vi "play-AFM-raster-imaging-open-loop.vi"() -> ()   [LabVIEW 2015]
uses:
  raster-scan-params.ctl
  <vilib>/userdefined/High Color/nirio_resource_hc.ctl
  <vilib>/Utility/file.llb/Read From Spreadsheet File (DBL).vi
  <vilib>/FPGAPlugInAG/cRIO-9082/niLvFpga_Open_cRIO-9082.vi
  <vilib>/rvi/interface/common/dynamic/niFpgaDynamicAddResources.vi
  <vilib>/FPGAPlugInAG/Dynamic/niLvFpga_Reset_Dynamic.vi
  <vilib>/rvi/interface/common/niFpgaWaitOnOcc.vi
  <vilib>/Utility/error.llb/Error Cluster From Error Code.vi
  <vilib>/rvi/errors/niLvFpgaAdjustHostInterfaceError.vi
  <vilib>/FPGAPlugInAG/Dynamic/niLvFpga_Run_Dynamic.vi
  <vilib>/Utility/file.llb/Write To Spreadsheet File (DBL).vi
  <vilib>/FPGAPlugInAG/Dynamic/niLvFpga_Close_Dynamic.vi
  <vilib>/rvi/interface/nirviOpenFPGA/nirviOpenFPGA.xnode
  FPGA Bitfiles/afmimagingcontro_FPGATargetSPARTA_raster-scanning_DXF4O8EAjZ4.lvbitx
  <vilib>/rvi/interface/nirviMethod/nirviMethod.xnode
  <vilib>/rvi/interface/nirviReadWriteControl/nirviReadWriteControl.xnode
  <vilib>/rvi/interface/nirviCloseFPGA/nirviCloseFPGA.xnode
  <vilib>/FPGAPlugInAG/Dynamic/niLvFpga_ConfigureFifo_Dynamic.vi
  <vilib>/rvi/errors/niLvFpgaMergeErrorWithErrorCode.vi
  <vilib>/rvi/interface/Simulation/niFpgaSimulationCallBeginRW.vi
  <vilib>/FPGAPlugInAG/Dynamic/niLvFpga_ReadFifo_Dynamic.vi
  NiFpgaLv.dll
  <vilib>/FPGAPlugInAG/Dynamic/niLvFpga_WriteFifo_Dynamic.vi
panel:
  out "Intensity Grapp":dbl[][](graph)
  in  "number-of-pixels":i32=256
  out "Waveform Graph 2":dbl[](graph)
  out "ramp-rate":sgl
  in  "points_per_line":i32=250000
  out "e(0) (threshhold init)":fxp<+/-,16,5>
  out "case-selector-feedback":i16
  in  "STOP":bool
  out "DAC-zaxis":sgl
  out "nsamps":i32
  in  "constant 2 lower":bool
  in  "raise-constant":sgl
  out "trigger":bool
  in  "raster-scan-params":T1={"TsTicks"=1600, "force setpoint"=0.0, "Stop"=FALSE, "Ki"=0.001, "TOL"=0.3, "ramp-rate"=1e-07, "z-u-max"=5.0} {"ramp-rate" format="%#_13g"; "TOL" format="%#_13g"}
  in  "raise-constant (init)":sgl
  out "Waveform Graph":dbl[](graph)
  out "ADC-zaxis":sgl
  out "elements left":i32=1
  in  "reference traj path":path=path "C:/Users/arnold/Documents/labview/afm_imaging/data/data-in-.csv"
  in  "outputData BOTH":path=path "C:/Users/arnold/Documents/labview/afm_imaging/data/data-out.csv"
  out "y iter":i32
  out "size(s)":i32
  in  "x_ffK":dbl=0.307692307692308 format="%#_13g"
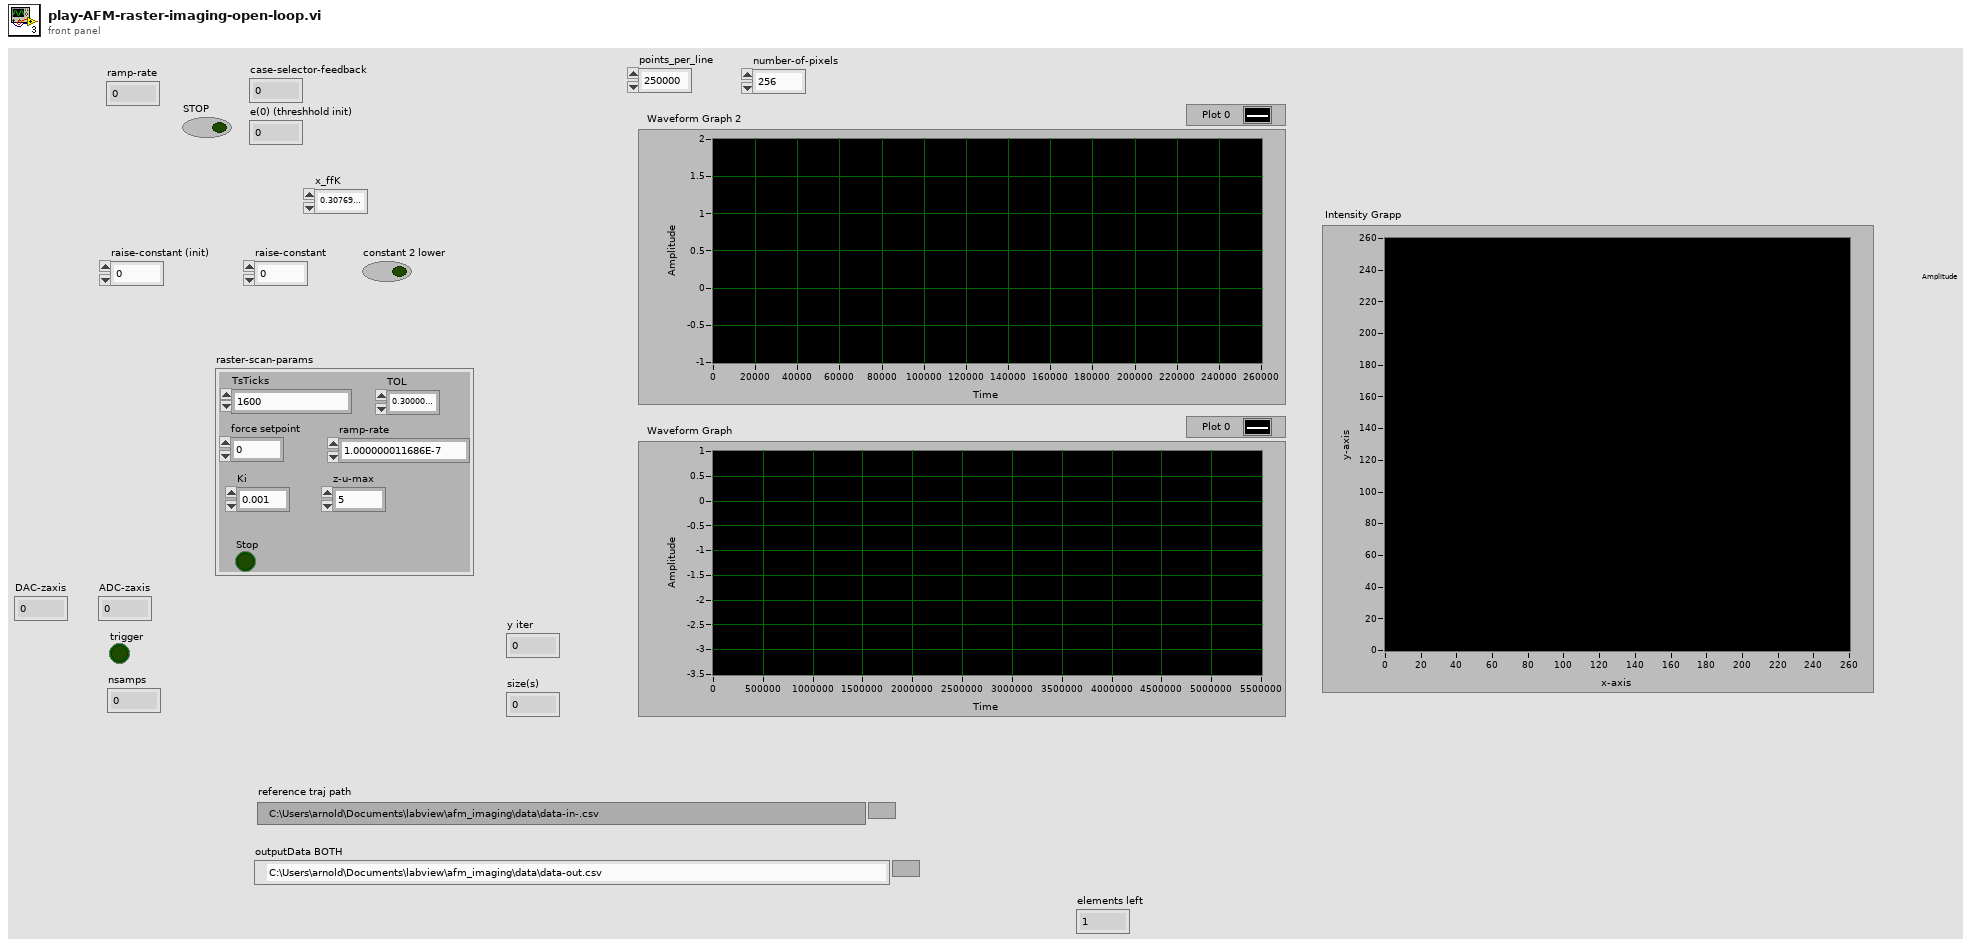
[diagram p1: front panel]
types:
  T1 = typedef "raster-scan-params.ctl" = cluster{"TsTicks":u32, "force setpoint":sgl, "Stop":bool, "Ki":sgl, "TOL":sgl, "ramp-rate":sgl, "z-u-max":sgl}
  T2 = typedef "nirio_resource_hc.ctl" = tag
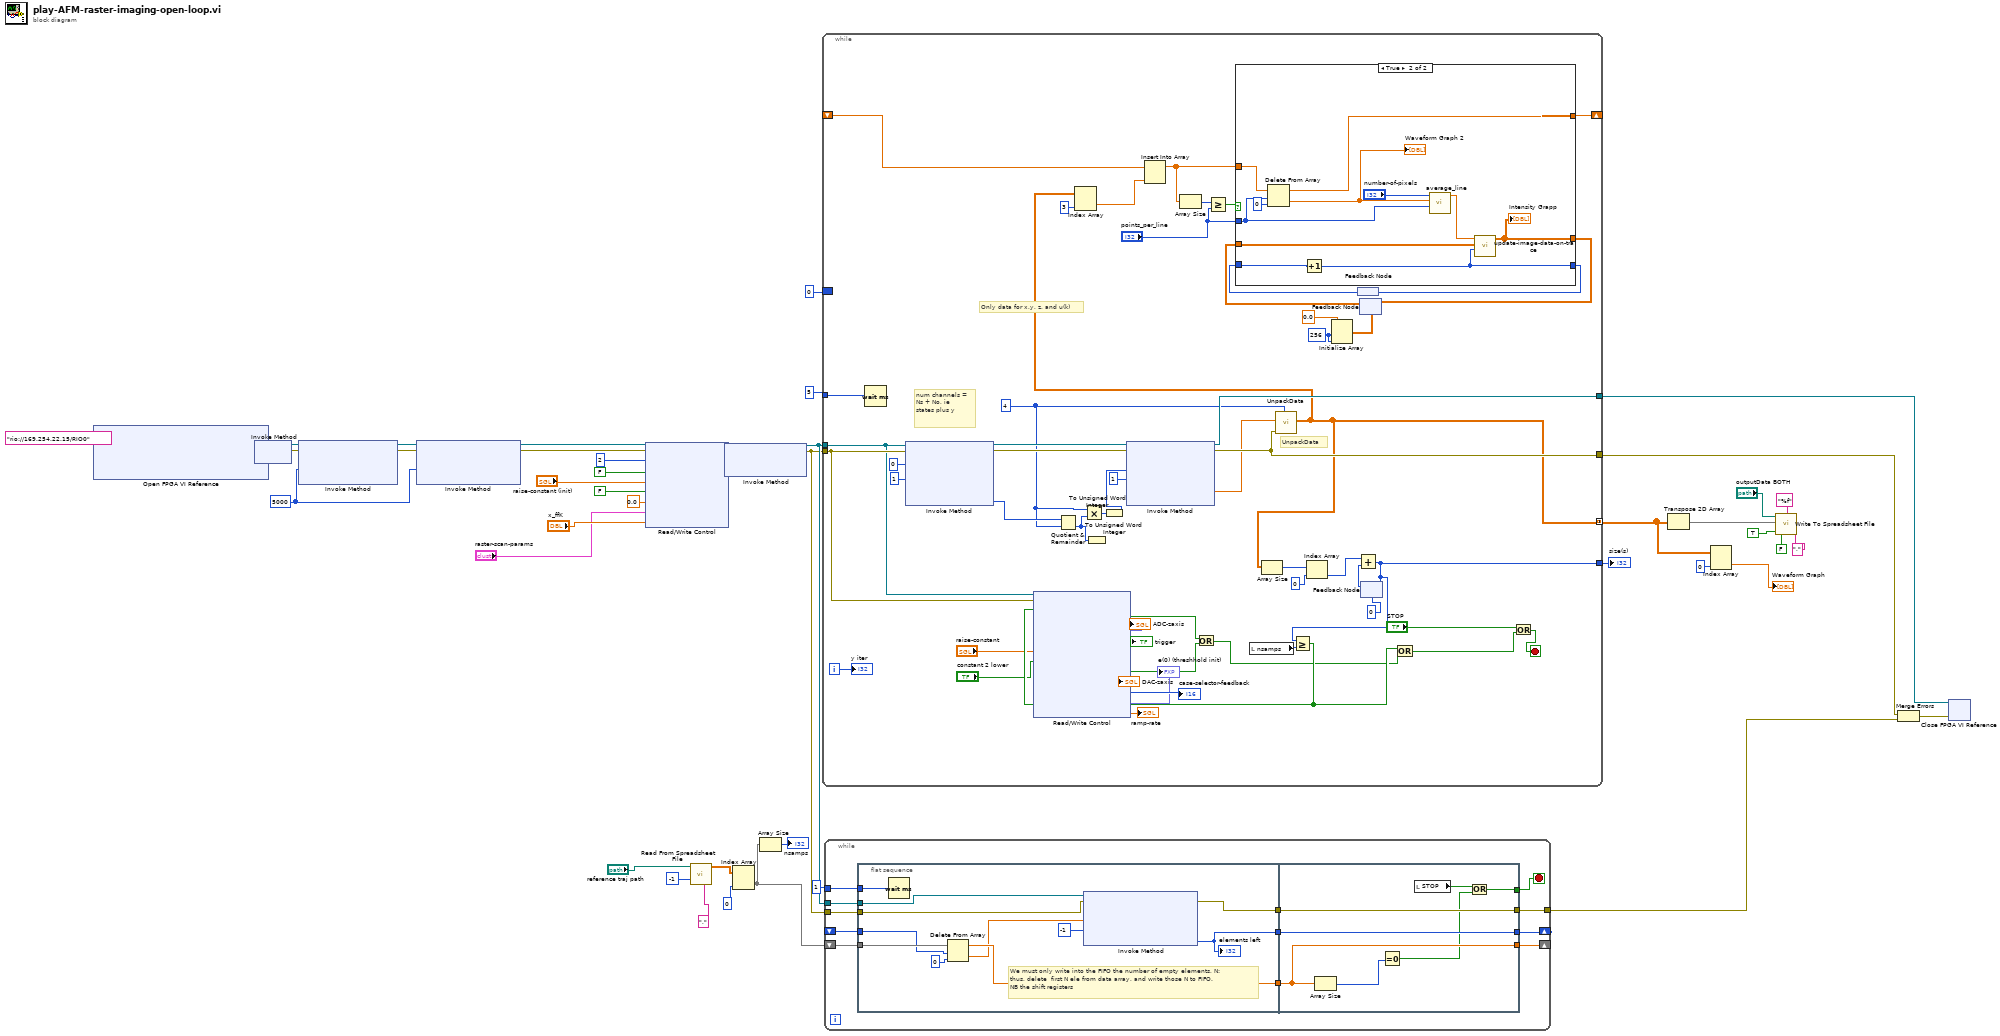
[diagram p0: block diagram]
diagram:
  w40 = 5000
  n1 = xnode "Open FPGA VI Reference"("resource name"=T2 "rio://169.254.22.15/RIO0") -> ("FPGA VI Reference Out"=w39:refnum<k20>, "error out"=w38:errorcluster)  [unwired: 1 in]
  n2 = xnode "Invoke Method"("FPGA VI Reference In"=w39, "error in"=w38) -> ("FPGA VI Reference Out"=w16:refnum<k20>, "error out"=w15:errorcluster)
  n3 = xnode "Invoke Method"("FPGA VI Reference In"=w16, "error in"=w15, "Requested Depth"=w40) -> ("FPGA VI Reference Out"=w20:refnum<k20>, "error out"=w21:errorcluster)  [unwired: 1 out]
  n4 = xnode "Invoke Method"("FPGA VI Reference In"=w20, "error in"=w21, "Requested Depth"=w40) -> ("FPGA VI Reference Out"=w42:refnum<k20>, "error out"=w41:errorcluster)  [unwired: 1 out]
  n5 = xnode "Read/Write Control"("FPGA VI Reference In"=w42, "error in"=w41, "initial case"=i16 2, "constant 2 lower"=FALSE, "raise-constant"="raise-constant (init)", "PID to tip up"=FALSE, "u(0)"=sgl 0.0, "raster-scan-params"="raster-scan-params", "x_ffK"="x_ffK") -> ("FPGA VI Reference Out"=w18:refnum<k20>, "error out"=w17:errorcluster)
  n6 = call-poly <vilib>:"Read From Spreadsheet File.vi"("delimiter (\\t)"=",", "number of rows (all:-1)"=-1, "file path (dialog if empty)"="reference traj path") -> ("all rows"=w27:dbl[][])  [unwired: 4 in, 4 out]
  n7 = xnode "Invoke Method"("FPGA VI Reference In"=w18, "error in"=w17) -> ("FPGA VI Reference Out"=w23:refnum<k20>, "error out"=w22:errorcluster)  [unwired: 1 in]
  n8 = Index Array(array=w27, index (col)=0 ("dimension size")) -> (element=w5:dbl[])  [unwired: 1 in]
  n9 = Array Size(array=w5) -> (size(s)=→"nsamps":i32)
  n10 = while {
    tunnel: 5 -> [w100]
    tunnel: w23 -> [w80]
    tunnel: w22 -> [w81]
    tunnel: [w92] -> w25
    tunnel: [w91] -> w44
    tunnel: [w62] -> w11 mode=concatenating
    tunnel: [w78] -> w43
    shift-right: [w60] -> _
    shift-left: _ -> [w58]
    border: 0 ("disabled index (col)") -> [_]
    i -> [w79]
    stop <- w66 stop-if-true
    w48 = 256 ("dimension size")
    w75 = u32 4 ("y")
    # "num channels = Ns + No, ie states plus y"
    # "Only data for x,y, z, and u(k)"
    # "UnpackData"
    n11 = Wait (ms)(milliseconds to wait=w100) -> ()  [unwired: 1 out]
    n12 = xnode "Invoke Method"("FPGA VI Reference In"=w80, "error in"=w81, "Number of Elements"=0 ("Timeout (ms)"), "Timeout (ms)"=1) -> ("FPGA VI Reference Out"=w96:refnum<k20>, "error out"=w97:errorcluster, "Elements Remaining"=w87:u32)  [unwired: 1 out]
    n13 = Quotient & Remainder(x=w87, y=w75) -> (floor(x/y)=w89:u32)  [unwired: 1 out]
    n14 = Multiply(x=w75, y=w89) -> (x*y=w94:u32)
    n15 = To Unsigned Word Integer(number=w89) -> ()  [unwired: 1 out]
    n16 = To Unsigned Word Integer(number=w94) -> (unsigned 16bit integer=w90:u16)
    n17 = xnode "Invoke Method"("FPGA VI Reference In"=w96, "error in"=w97, "Number of Elements"=w90, "Timeout (ms)"=1) -> ("FPGA VI Reference Out"=w91:refnum<k20>, "error out"=w92:errorcluster, "Data"=w86:sgl[])  [unwired: 1 out]
    n18 = local read "nsamps"() -> (w88:i32)
    n19 = call "UnpackData.vi"("NumChannels"=w75, "error In"=w92, "1D Data In"=w86) -> ("2D Data Out"=w62:dbl[][])  [unwired: 7 in, 1 out]
    n20 = Index Array(array=w62, index (col)=3 ("disabled index (col)")) -> (element=w57:dbl[])  [unwired: 1 in]
    n21 = Insert Into Array(array=w58, new element=w57) -> (w55:dbl[])  [unwired: 1 in]
    n22 = Array Size(array=w55) -> (size(s)=w59:i32)
    n23 = Greater Or Equal?(x=w59, y="points_per_line") -> (x >= y?=w56:bool)
    n24 = Array Size(array=w62) -> (size(s)=w85:i32[])
    n25 = Index Array(array=w85, index=0) -> (element=w83:i32)
    n26 = Initialize Array(0.0 ("element"), w48, w48) -> (w46:dbl[][])
    n27 = feedback #1() -> (w49:i32)
    n28 = feedback #2(w46) -> (w51:dbl[][])
    n29 = case shown="True" w56 {
      tunnel: [w103 w112] -> w60
      tunnel: w55 -> [w103 w114]
      tunnel: "points_per_line" -> [_ w109]
      tunnel: [w102 w104] -> w52
      tunnel: w51 -> [w102 w107]
      tunnel: w49 -> [w101 w106]
      tunnel: [w101 w105] -> w50
      frame False {
      }
      frame True {
        n30 = Delete From Array(array=w114, length=w109, index=0) -> (deleted portion=w110:dbl[], array with subset deleted=w112:dbl[])
        "Waveform Graph 2" <- w110
        n31 = Increment(x=w106) -> (x+1=w105:i32)
        n32 = call "average_line.vi"("data-pts-per-line"=w109, "raw-data-row"=w110, "number-of-pixels"="number-of-pixels") -> ("avg-data-row"=w108:dbl[])  [unwired: 8 in]
        n33 = call "update-image-data-on-trace.vi"("iterator"=w105, "master-image-data-n"=w107, "avg-data-row"=w108) -> ("master-image-data-out"=w104:dbl[][])  [unwired: 8 in]
        "Intensity Grapp" <- w104
      }
    }
    n34 = feedback-in #1(w50) -> ()
    n35 = feedback-in #2(w52) -> ()
    n36 = feedback #3(0) -> (w84:i32)
    n37 = Add(x=w83, y=w84) -> (x+y=w78:i32)
    n38 = Greater Or Equal?(x=w78, y=w88) -> (x >= y?=w76:bool)
    n39 = xnode "Read/Write Control"("FPGA VI Reference In"=w80, "error in"=w81, "PID to tip up"=w76, "raise-constant"="raise-constant", "constant 2 lower"="constant 2 lower") -> ("unstable-traj"=w70:bool, "ADC-zaxis"=→"ADC-zaxis":fxp<+/-,24,5>, "trigger"=→"trigger":bool, "scanning-finished"=w69:bool, "DAC-zaxis"=→"DAC-zaxis":sgl, "case-selector-feedback"=→"case-selector-feedback":i16, "e(0) (threshhold init)"=→"e(0) (threshhold init)":fxp<+/-,16,5>, "ramp-rate"=→"ramp-rate":sgl)  [unwired: 2 out]
    n40 = Or(x=w70, y=w69) -> (x .or. y?=w71:bool)
    n41 = feedback-in #3(w78) -> ()
    n42 = Or(x=w76, y=w71) -> (x .or. y?=w67:bool)
    n43 = Or(x="STOP", y=w67) -> (x .or. y?=w66:bool)
    "y iter" <- w79
  }
  "size(s)" <- w43
  n44 = while {
    tunnel: [w124] -> w19
    tunnel: 1 -> [w126]
    shift-right: [w120] -> _
    shift-left: _ -> [w123]
    shift-right: [w118] -> _
    shift-left: w5 -> [w125]
    tunnel: w23 -> [w117]
    tunnel: w22 -> [w116]
    stop <- w115 stop-if-true
    n45 = flat-sequence {
      tunnel: w126 -> [w137]
      tunnel: w125 -> [w132]
      tunnel: w123 -> [w128]
      tunnel: [w135] -> w122
      tunnel: [w133] -> w121
      tunnel: [w134] -> w119
      tunnel: w117 -> [w130]
      tunnel: w116 -> [w129]
      tunnel: [w144] -> w120
      tunnel: [w141] -> w124
      tunnel: w122 -> [w141]
      tunnel: w121 -> [w144]
      tunnel: w119 -> [w142]
      tunnel: [w142] -> w118
      tunnel: [w138] -> w115
      frame #0 {
        # "We must only write into the FIFO the number of empty elements, N:\nthus, delete  first N ele from data array, and write those N to FIFO.\nNB the shift registers"
        n46 = Wait (ms)(milliseconds to wait=w137) -> ()  [unwired: 1 out]
        n47 = Delete From Array(array=w132, length=w128, index=0) -> (deleted portion=w131:dbl[], array with subset deleted=w134:dbl[])
        n48 = xnode "Invoke Method"("FPGA VI Reference In"=w130, "error in"=w129, "Data"=w131, "Timeout (ms)"=-1) -> ("error out"=w135:errorcluster, "Empty Elements Remaining"=w133:u32)  [unwired: 1 out]
        "elements left" <- w133
      }
      frame #1 {
        n49 = Array Size(array=w142) -> (size(s)=w143:i32)
        n50 = Equal To 0?(x=w143) -> (x = 0?=w140:bool)
        n51 = local read "STOP"() -> (w139:bool)
        n52 = Or(x=w139, y=w140) -> (x .or. y?=w138:bool)
      }
    }
  }
  n53 = Transpose 2D Array(2D array=w11) -> (transposed array=w14:dbl[][])
  n54 = Index Array(array=w11, index (col)=0 ("disabled index (col)")) -> (element=→"Waveform Graph":dbl[])  [unwired: 1 in]
  n55 = call-poly <vilib>:"Write To Spreadsheet File.vi"("delimiter (\\t)"=",", "transpose? (no:F)"=TRUE, "format (%.3f)"="%f", "append to file? (new file:F)"=FALSE, "2D data"=w14, "file path (dialog if empty)"="outputData BOTH") -> ()  [unwired: 2 in, 1 out]
  n56 = Merge Errors(w25, w19) -> (w24:errorcluster)
  n57 = xnode "Close FPGA VI Reference"("FPGA VI Reference In"=w44, "error in"=w24) -> ()  [unwired: 1 out]
